vi "PH_Beckhoff_PP_PU.get Instance from PU.vi"(1 "PU":T1) -> (0 "Beckhoff PU Instance":string)   [LabVIEW 2014, in "PH_Beckhoff_PP_PU.lvlib"]
uses:
  PH_Beckhoff_PP_PU.lvlib
  PH_Basics/PH_PP_Common/PH_PP_Common.PUs.ctl
  PH_Basics/PH_PP_Common/PH_PP_Common.lvlib
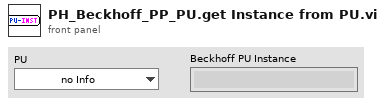
[diagram p1: front panel]
types:
  T1 = typedef "PH_PP_Common.lvlib/PH_PP_Common.PUs.ctl" = enum16{"no Info", "PA-19mm-1", "PA-19mm-2", "PA-45mm-PILC", "PA-45mm-MAIN", "MA-PU-1", "MA-PU-2", "MA-PU-3", "MA-PU-4", "MA-PU-5", "MA-PU-6", "MA-FR", "MA-PILC", "PA-45mm-DP"}
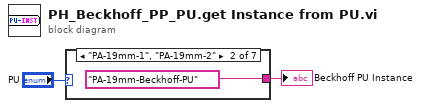
[diagram p0: block diagram]
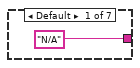
[diagram p2: hidden frame]
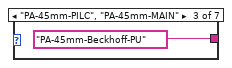
[diagram p3: hidden frame]
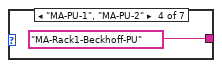
[diagram p4: hidden frame]
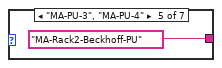
[diagram p5: hidden frame]
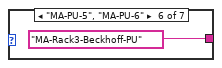
[diagram p6: hidden frame]
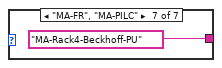
[diagram p7: hidden frame]
diagram:
  n1 = case shown="\"PA-19mm-1\", \"PA-19mm-2\"" "PU" {
    tunnel: ["N/A" "PA-19mm-Beckhoff-PU" "PA-45mm-Beckhoff-PU" "MA-Rack1-Beckhoff-PU" "MA-Rack2-Beckhoff-PU" "MA-Rack3-Beckhoff-PU" "MA-Rack4-Beckhoff-PU"] -> w1
    frame Default {
    }
    frame "PA-19mm-1", "PA-19mm-2" {
    }
    frame "PA-45mm-PILC", "PA-45mm-MAIN" {
    }
    frame "MA-PU-1", "MA-PU-2" {
    }
    frame "MA-PU-3", "MA-PU-4" {
    }
    frame "MA-PU-5", "MA-PU-6" {
    }
    frame "MA-FR", "MA-PILC" {
    }
  }
  "Beckhoff PU Instance" <- w1
